vi "Main.vi"() -> ()   [LabVIEW 2020]
doc: "[Covers: REQ08]\n[Covers: REQ04]\n[Covers: REQ05]\n[Covers: REQ01]\n[Covers: REQ07]\n[Covers: REQ11]\n[Covers: REQ13]\n[Covers: REQ14]\n[Covers: REQ16]\n[Covers: REQ17]\n[Covers: REQ18]\n[Covers: REQ19]\n[Covers: REQ02]\n[Covers: REQ20]\n[Covers: REQ21]"
uses:
  TypeDef's/Estados - Consumidor.ctl
  TypeDef's/Dados consumidor.ctl
  <vilib>/Utility/sysdir.llb/System Directory Type.ctl
  <vilib>/Waveform/WDTOps.llb/WDT Append Waveforms DBL.vi
  <vilib>/Waveform/WDTOps.llb/WDT Waveform Duration DBL.vi
  <vilib>/measure/NI_MABase.lvlib
panel:
  in  "physical channels":tag
  in  "Canal físico":tag
  in  "Boolean 2":bool
  in  "Boolean":bool
  in  "Power":bool
  in  "Concatenar":bool
  in  "Adquirir entre cursores":bool
  in  "Deletar entre cursores":bool
  in  "Concatenar entre cursores":bool
  in  "Fase         º":dbl(slide) caption="Horizontal Slider" min=0.0 max=360.0 step=0.5 scale=0.0..360.0 scale format="%#.6g"
  in  "Offset":dbl(slide) caption="Vertical Slider" min=-10.0 max=10.0 step=0.01 scale=-10.0..10.0 scale format="%#2_2g"
  in  "Forma de onda":T1(ring) caption="Enum"
  in  "Tempo (Segundos)":dbl(knob)=1.0 min=0.0 max=1.0 step=0.01 scale=0.0..1.0
  in  "Abrir arquivo":bool
  in  "Salvar":bool
  out "Edição":waveform(dbl)(graph)
  out "Plot":waveform(dbl)(graph)
  in  "Razão cíclica (%)":dbl(knob)=50.0 min=0.0 max=100.0 step=0.5 scale=0.0..100.0
  in  "Amplitude":dbl(knob)=5.0 min=0.0 max=10.0 step=0.01 scale=0.0..10.0
  in  "Frequência":dbl(knob)=1.0 min=0.0 max=10.0 step=0.01 scale=0.0..10.0
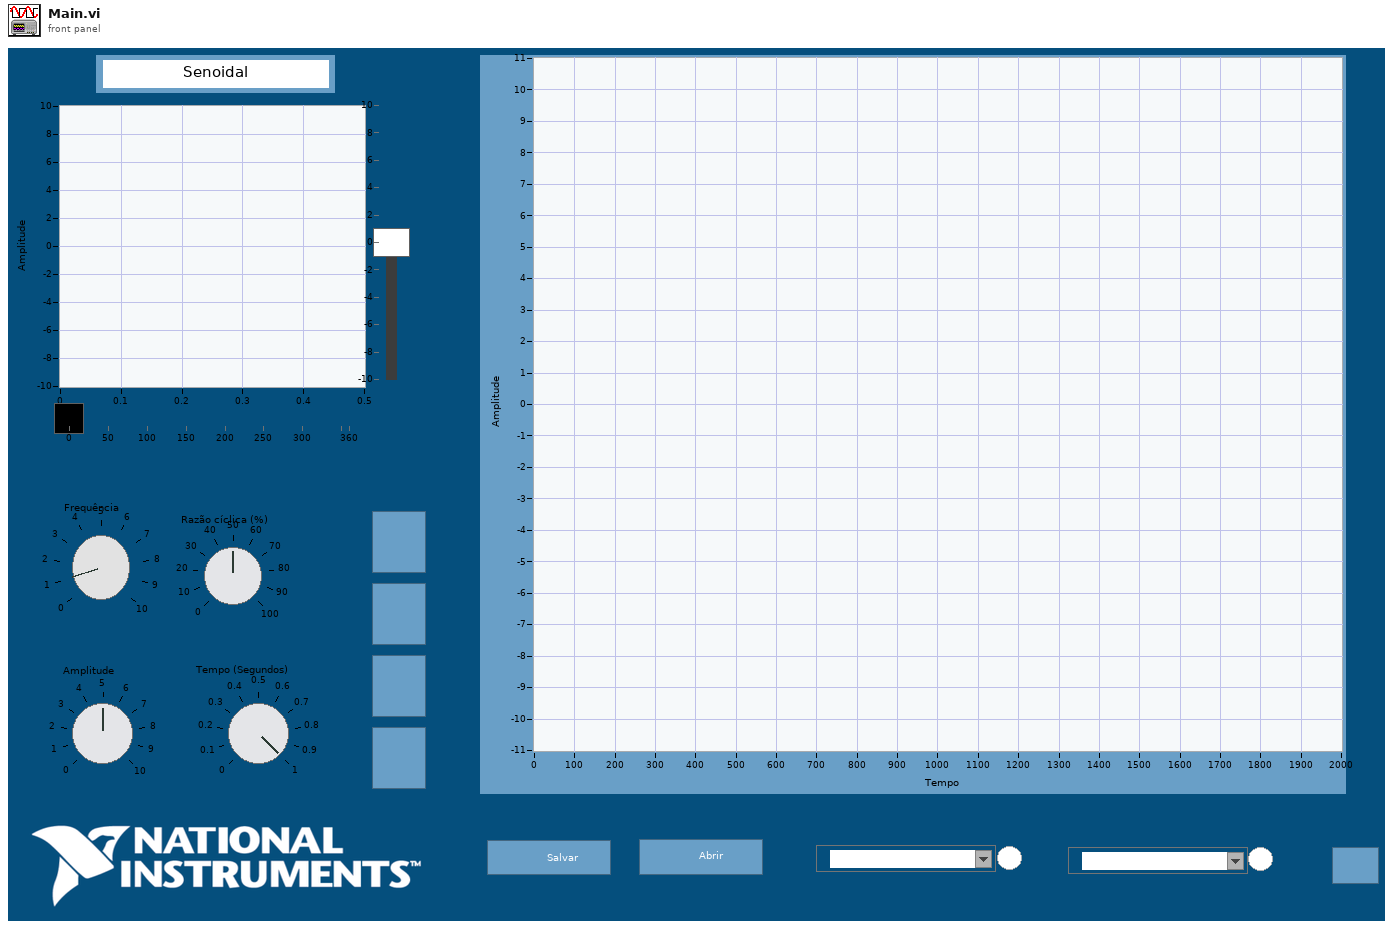
[diagram p1: front panel]
types:
  T1 = enum16{"Senoidal", "Triangular", "Quadrada", "Dente de Serra", "Trapezoidal"}
  T2 = enum16{"create", "fire - Simular onda", "fire - Editar onda", "fire - Salvar ou carregar onda", "destroy"}
  T3 = typedef "Estados - Consumidor.ctl" = enum16{"Gerar onda", "Inicialização", "Parada", "Plotar", "Concatenar", "Concatenar - Cursores", "Adquirir entre Cursores", "Deletar entre Cursores", "Salvar onda", "Carregar onda", "Posicionar Cursores", "Atualizar controles - Servidor", "Enviar onda - hardware", "Ler onda - hardware"}
  T4 = typedef "Dados consumidor.ctl" = cluster{"Onda gerada":cluster{"onda":waveform(dbl)}, "Onda modificada":cluster{"onda":waveform(dbl)}, "task out":refnum<k21>}
  T5 = typedef "Informações.ctl" = cluster{"Estados":T3, "Amplitude":dbl, "Informação\nde amostragem":cluster{"Fs":dbl, "#s":dbl}, "Frequência":dbl, "Offset":dbl, "Fase (Graus)":dbl, "Razão cíclica (%)":dbl, "Sinal":enum16{"Sine Wave", "Triangle Wave", "Square Wave", "Sawtooth Wave", "Trapezoidal Wave"}, "event registration refnum":refnum<event-registration>, "Posição Cursor 0":dbl, "Posição Cursor 1":dbl, "Flag Edição":i32}
  T6 = enum8{"Enabled", "Disabled", "Disabled and Grayed Out"}
  T7 = enum16{"Sine Wave", "Triangle Wave", "Square Wave", "Sawtooth Wave", "Trapezoidal Wave"}
  T8 = enum16{"open", "open or create", "create or replace", "create", "open (read-only)"}
  T9 = typedef "System Directory Type.ctl" = i32
  T10 = cluster{"Amostras / s":dbl, "Quantidade\nde amostras":dbl}
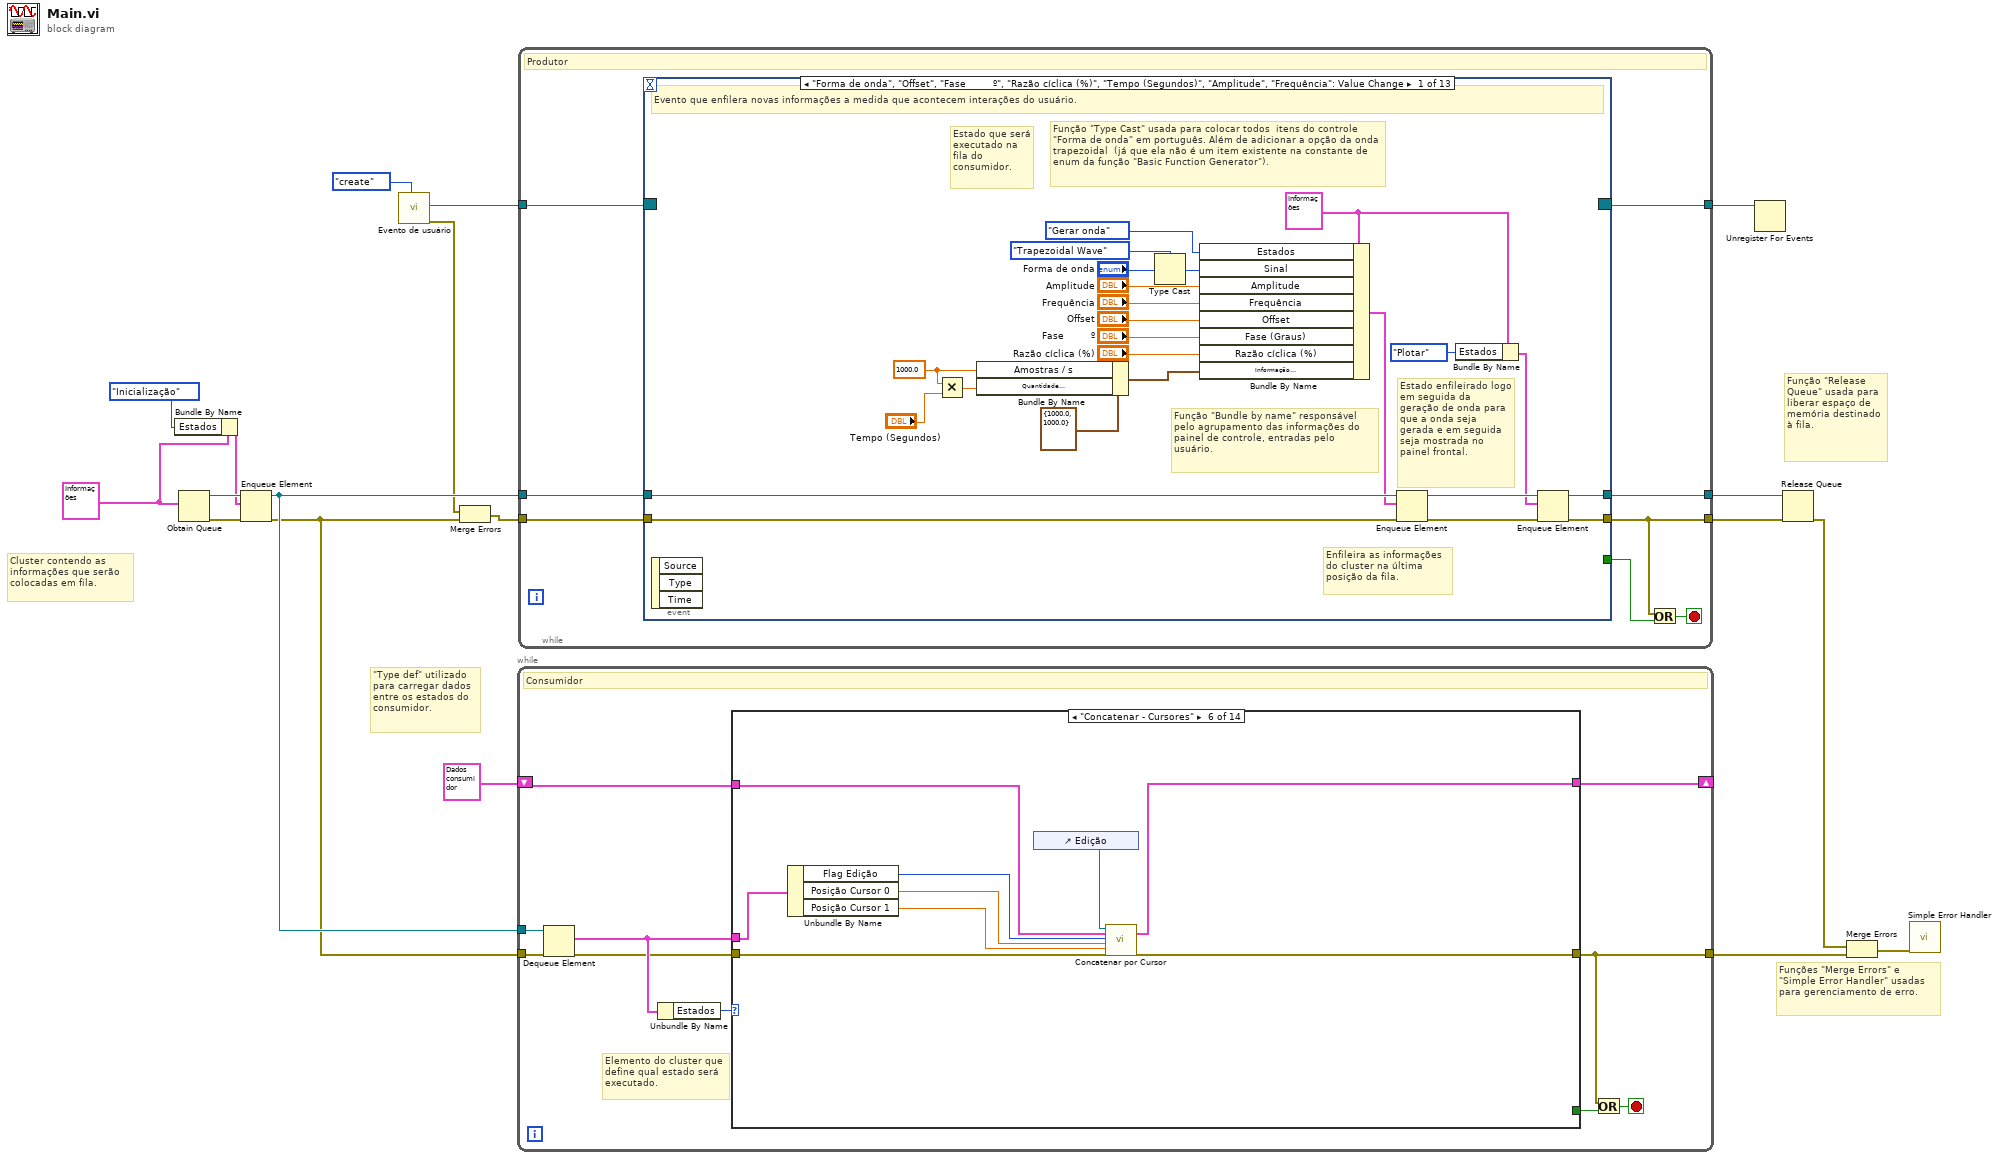
[diagram p0: block diagram]
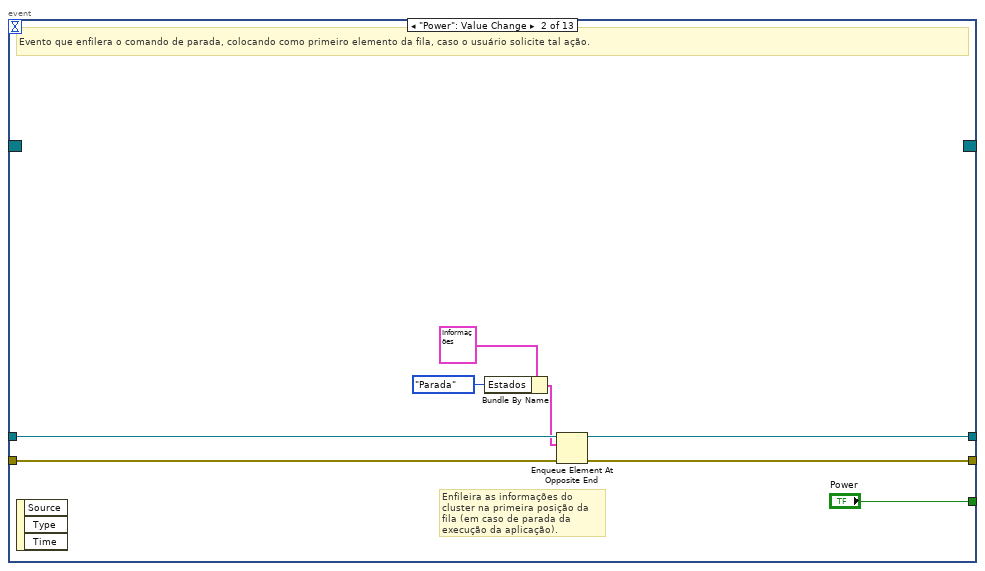
[diagram p2: hidden frame]
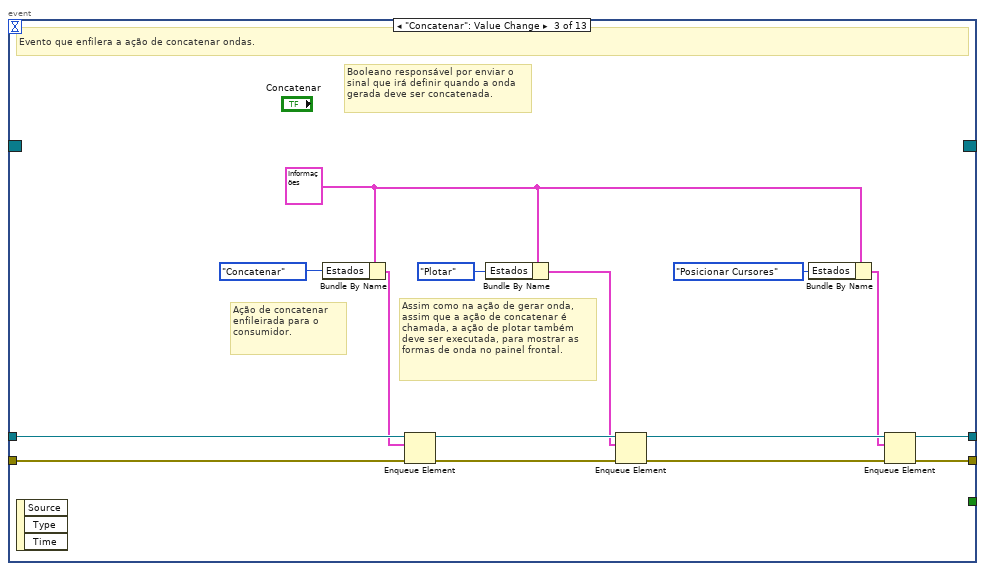
[diagram p3: hidden frame]
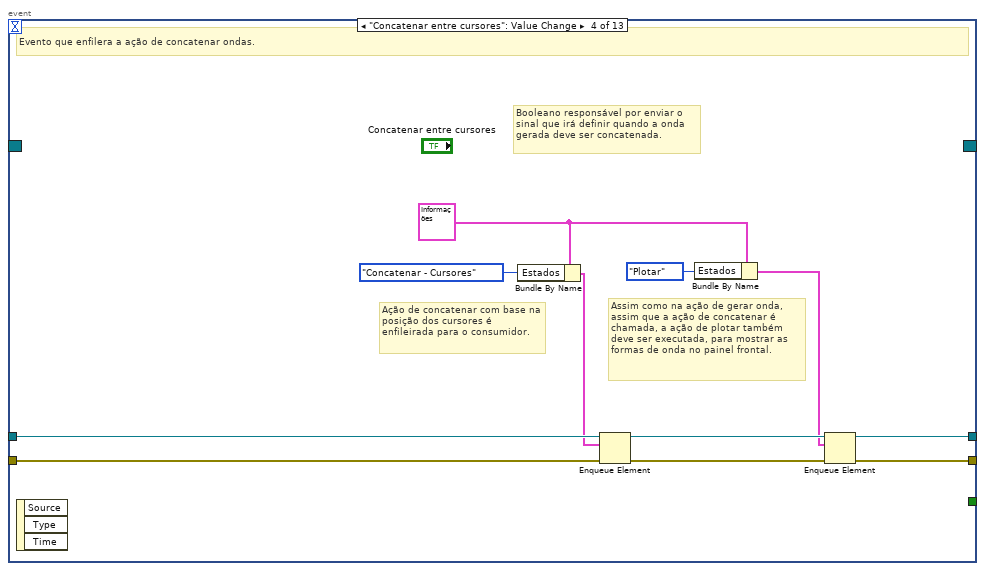
[diagram p4: hidden frame]
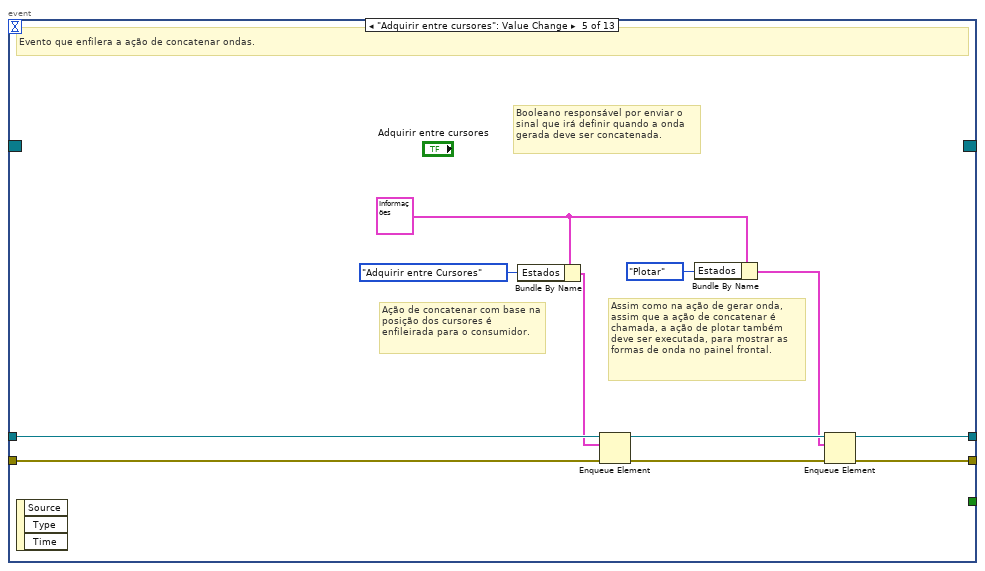
[diagram p5: hidden frame]
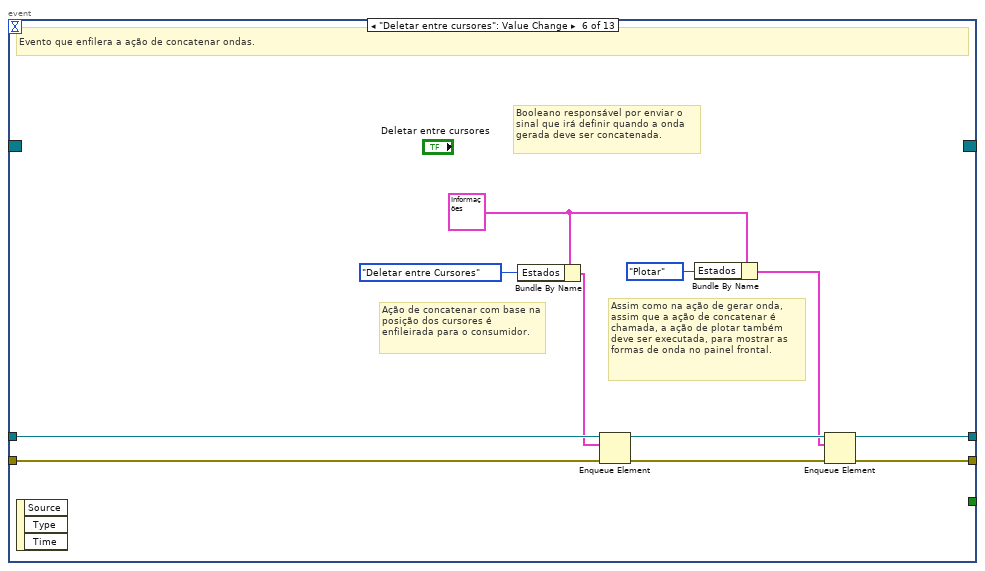
[diagram p6: hidden frame]
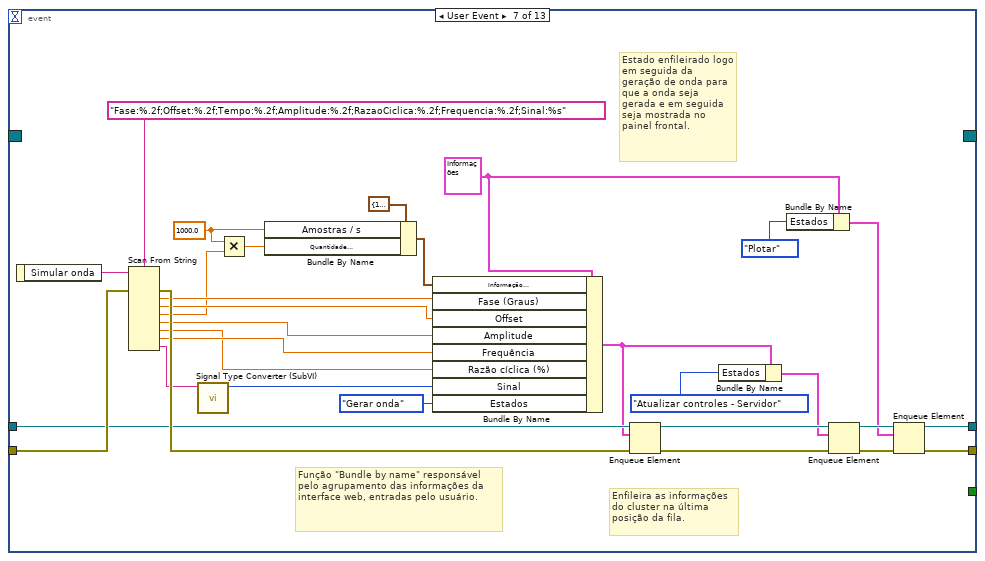
[diagram p7: hidden frame]
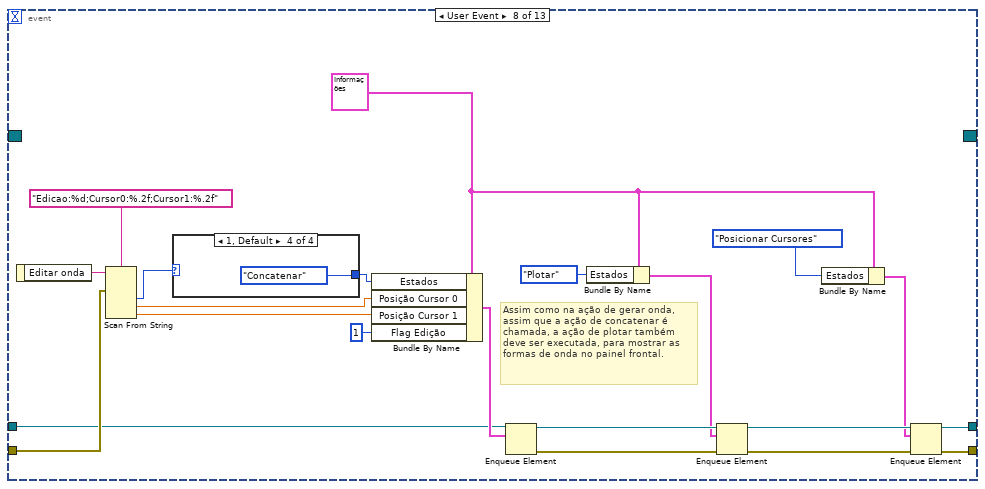
[diagram p8: hidden frame]
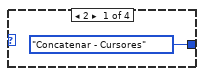
[diagram p9: hidden frame]
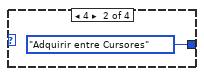
[diagram p10: hidden frame]
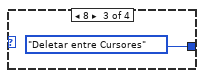
[diagram p11: hidden frame]
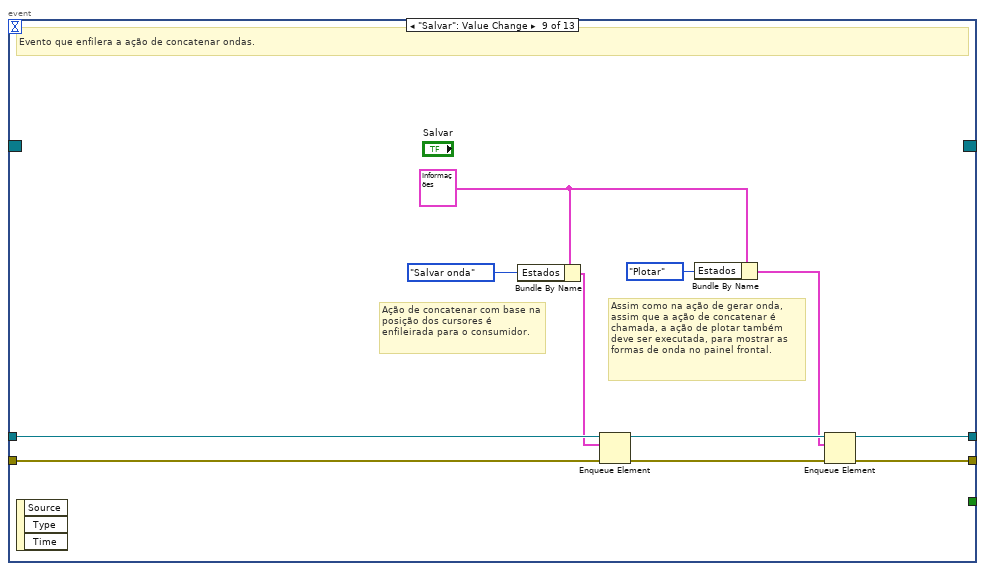
[diagram p12: hidden frame]
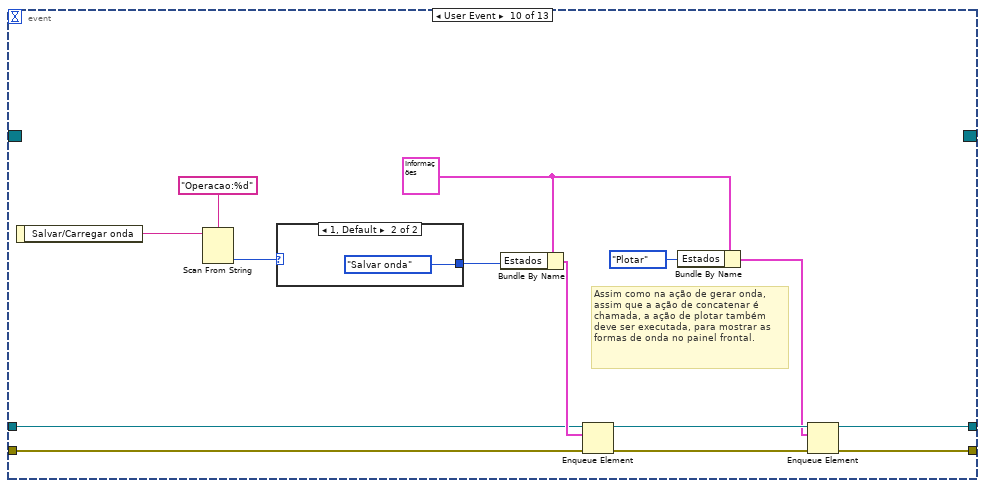
[diagram p13: hidden frame]
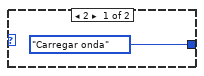
[diagram p14: hidden frame]
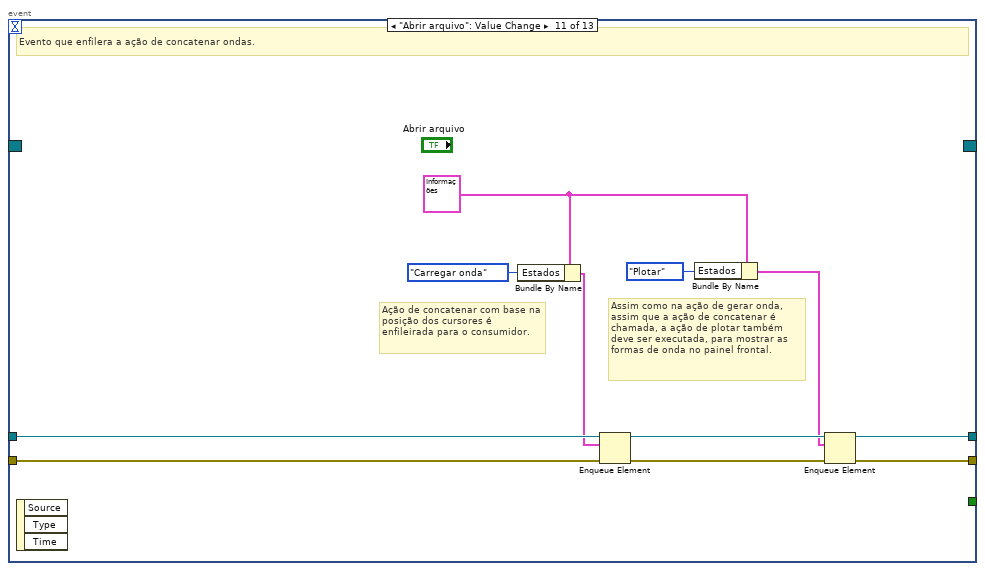
[diagram p15: hidden frame]
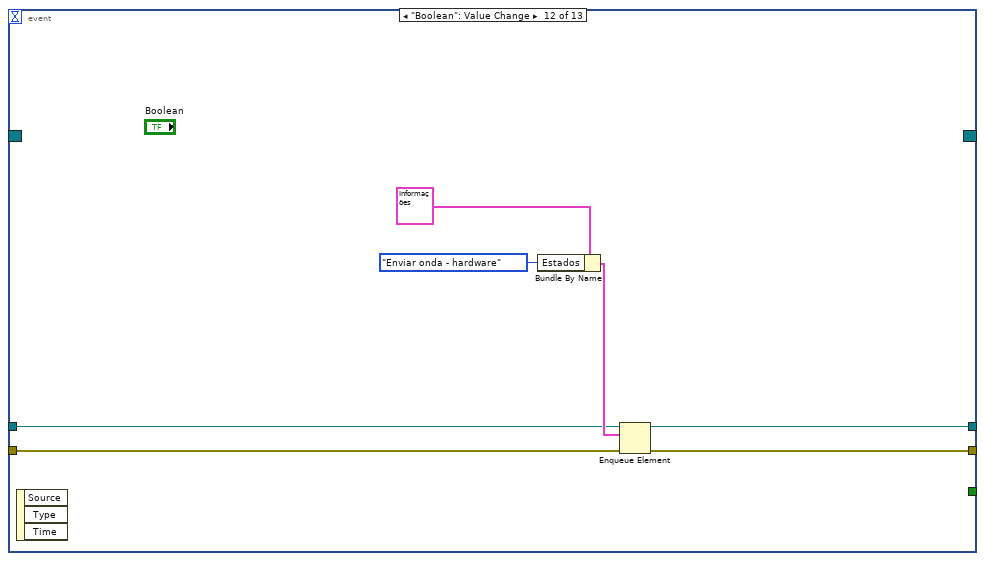
[diagram p16: hidden frame]
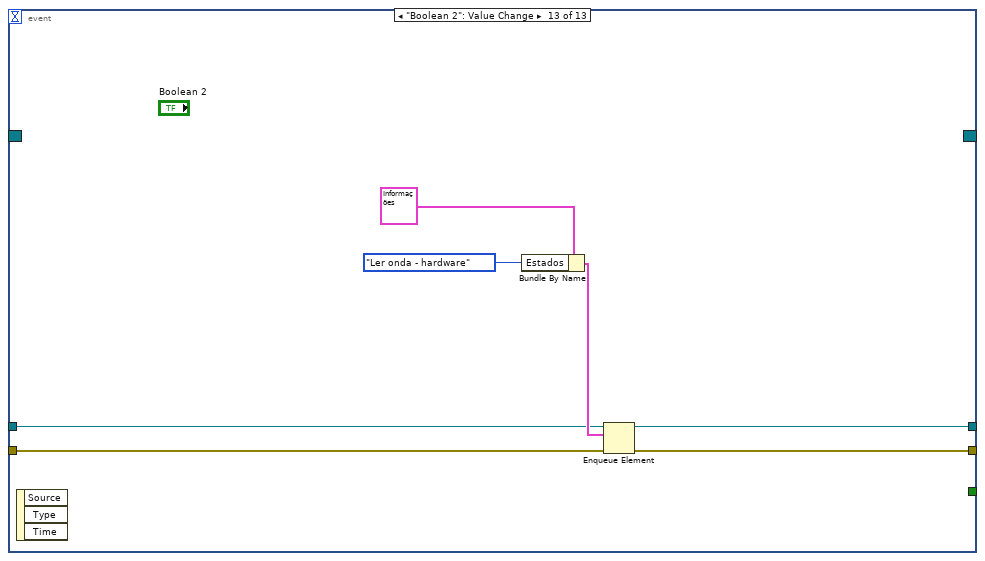
[diagram p17: hidden frame]
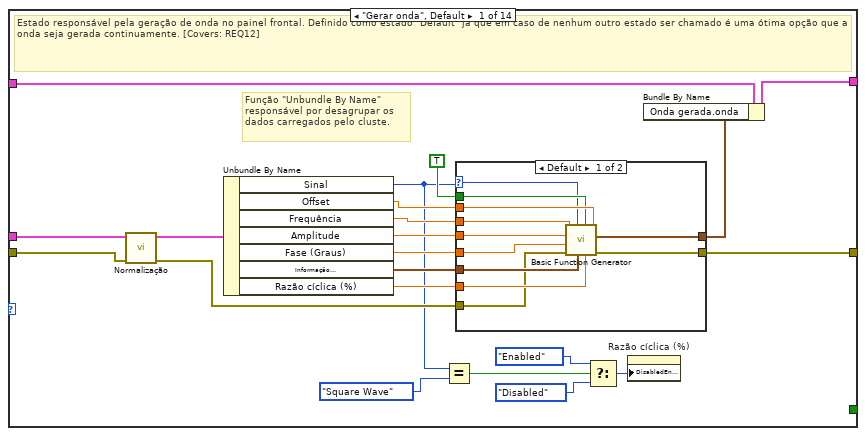
[diagram p18: hidden frame]
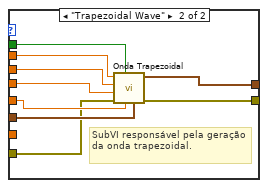
[diagram p19: hidden frame]
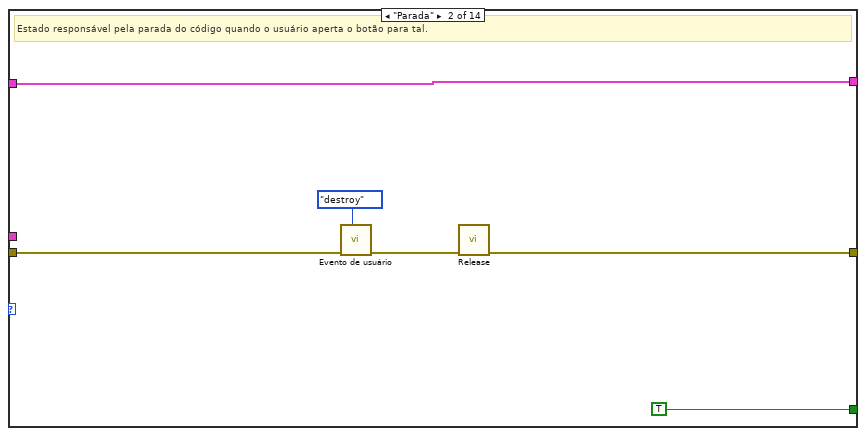
[diagram p20: hidden frame]
diagram:
  w7 = T5 {"Estados"=enum."Gerar onda", "Amplitude"=0.0, "Informação\nde amostragem"={"Fs"=1000.0, "#s"=1000.0}, "Frequência"=0.0, "Offset"=0.0, "Fase (Graus)"=0.0, "Razão cíclica (%)"=0.0, "Sinal"=enum."Sine Wave", "event registration refnum"=refnum, "Posição Cursor 0"=0.0, "Posição Cursor 1"=0.0, "Flag Edição"=0}
  # "\"Type def\" utilizado para carregar dados entre os estados do consumidor."
  # "Funções \"Merge Errors\" e \"Simple Error Handler\" usadas para gerenciamento de erro."
  # "Função \"Release Queue\" usada para liberar espaço de memória destinado à fila."
  # "Cluster contendo as informações que serão colocadas em fila."
  n1 = Bundle By Name(cluster=w7, "Estados"=Estados_-_Consumidor."Inicialização") -> (w9:T5)
  n2 = Obtain Queue(element data type=w7) -> (queue out=w11:refnum<queue>, error out=w13:errorcluster)  [unwired: 4 in, 1 out]
  n3 = Enqueue Element(queue=w11, element=w9, error in (no error)=w13) -> (queue out=w10:refnum<queue>, error out=w6:errorcluster)  [unwired: 1 in, 1 out]
  n4 = call "Evento de usuário.vi"("Enum"=T2."create") -> ("error out"=w4:errorcluster, "Event Registration Refnum"=w3:refnum<event-registration>)  [unwired: 9 in]
  n5 = Merge Errors(w4, w6) -> (w5:errorcluster)
  n6 = while {
    tunnel: w10 -> [w22]
    tunnel: [w19] -> w15
    tunnel: w6 -> [w23]
    shift-right: [w21] -> _
    shift-left: T4 {"Onda gerada"={"onda"={"t0"=timestamp(0 s since 1904-01-01), "dt"=1.0, "Y"=[]}}, "Onda modificada"={"onda"={"t0"=timestamp(0 s since 1904-01-01), "dt"=1.0, "Y"=[]}}, "task out"=""} ("Cluster 3") -> [w20]
    stop <- w25 stop-if-true
    # "Elemento do cluster que define qual estado será executado."
    # "Consumidor"
    n7 = Dequeue Element(queue=w22, error in (no error)=w23) -> (element=w27:T5, error out=w24:errorcluster)  [unwired: 1 in, 2 out]
    n8 = Unbundle By Name(w27) -> ("Estados"=w28:T3)
    n9 = case shown="\"Concatenar - Cursores\"" w28 {
      tunnel: w27 -> [w49 _ _ _ _ w101 w110 w119 _ _ _ w204 _ _]
      tunnel: [_ TRUE _ _ _ _ _ _ _ _ _ _ _ _] -> w26
      tunnel: [w41 w70 w77 w84 w91 w105 w112 w123 w131 w152 w185 w193 w206 w225] -> w19
      tunnel: w24 -> [w36 w73 w82 w87 w91 w106 w113 w124 w127 w155 w188 w193 w211 w228]
      tunnel: [w39 w74 w83 w89 w92 w104 w111 w122 w128 w153 w190 w205 w212 w220] -> w21
      tunnel: w20 -> [w40 w74 w83 w90 w92 w102 w114 w121 w132 w154 w190 w205 w212 w220]
      frame "Gerar onda", Default {
        # "Função \"Unbundle By Name\" responsável por desagrupar os dados carregados pelo cluste."
        # "Estado responsável pela geração de onda no painel frontal. Definido como estado \"Default\" já que em caso de nenhum outro estado ser chamado é uma ótima opção que a onda seja gerada continuamente. [Covers: REQ12]"
        n10 = call "Normalização.vi"("error in (no error)"=w36, 11:w49) -> ("error out"=w35:errorcluster, 3:w37:T5)  [unwired: 8 in]
        n11 = Unbundle By Name(w37) -> ("Sinal"=w29:T7, "Offset"=w48:dbl, "Frequência"=w47:dbl, "Amplitude"=w46:dbl, "Fase (Graus)"=w45:dbl, "Informação\nde amostragem"=w44:cluster{"Fs":dbl, "#s":dbl}, "Razão cíclica (%)"=w43:dbl)
        n12 = Equal?(x=w29, y=T7."Square Wave" ("Sinal")) -> (x = y?=w34:bool)
        n13 = case shown="Default" w29 {
          selector: w29 -> [w52 _]
          tunnel: w48 -> [w60 w63]
          tunnel: w47 -> [w59 w65]
          tunnel: w46 -> [w58 w64]
          tunnel: w45 -> [w57 w68]
          tunnel: w44 -> [w56 w67]
          tunnel: w43 -> [w55 _]
          tunnel: [w54 w66] -> w38
          tunnel: TRUE ("reset signal") -> [w53 w69]
          tunnel: [w51 w61] -> w41
          tunnel: w35 -> [w50 w62]
          frame Default {
            n14 = call <vilib>:"Basic Function Generator.vi"("offset"=w60, "square wave duty cycle (%)"=w55, "reset signal"=w53, "sampling info"=w56, "signal type"=w52, "error in (no error)"=w50, "phase"=w57, "amplitude"=w58, "frequency"=w59) -> ("error out"=w51:errorcluster, "signal out"=w54:waveform(dbl))  [unwired: 1 out]
          }
          frame "Trapezoidal Wave" {
            # "SubVI responsável pela geração da onda trapezoidal."
            n15 = call "Onda Trapezoidal.vi"("Informação\nde amostragem"=w67, "Fase (Graus)"=w68, "Reset do sinal"=w69, "Entrada de erro"=w62, "Amplitude"=w64, "Frequência"=w65, "Offset"=w63) -> ("Saída de erro"=w61:errorcluster, "Saída de sinal"=w66:waveform(dbl))  [unwired: 3 in]
          }
        }
        n16 = Select(t=T6."Enabled" ("Disabled"), s=w34, f=T6."Disabled" ("Disabled")) -> (s? t:f=w33:T6)
        n17 = property on="Razão cíclica (%)" class="Knob (strict)"("DisabledEnum"=w33) -> ()  [unwired: 2 in, 2 out]
        n18 = Bundle By Name(cluster=w40, "Onda gerada.onda"=w38) -> (w39:T4)
      }
      frame "Parada" {
        # "Estado responsável pela parada do código quando o usuário aperta o botão para tal."
        n19 = call "Evento de usuário.vi"("Enum"=T2."destroy", "error in (no error)"=w73) -> ("error out"=w71:errorcluster)  [unwired: 8 in, 1 out]
        n20 = call "Release.vi"("error in"=w71) -> ("error out"=w70:errorcluster)  [unwired: 10 in]
      }
      frame "Plotar" {
        # "FGV responsável por atualizar os dados da onda para envio para a interface web"
        # "Plot da onda editada pelo usuário."
        # "Plot da onda definida e gerada pelo usuário."
        # "Estado encarregado de exibir no painel frontal as formas de onda."
        n21 = Unbundle By Name(w83) -> ("Onda gerada.onda"=w81:waveform(dbl))
        "Plot" <- w81
        n22 = call "Plotar gráficos.vi"("Enum"=enum16{"set", "get"}."set", "error in (no error)"=w82, "Entrada Cluster de onda"=w81) -> ("error out"=w78:errorcluster)  [unwired: 7 in, 1 out]
        n23 = Unbundle By Name(w83) -> ("Onda modificada.onda"=w76:waveform(dbl))
        "Edição" <- w76
        n24 = call "Plotar gráfico edição.vi"("Enum"=enum16{"set", "get"}."set", "error in (no error)"=w78, "Entrada Cluster de onda"=w76) -> ("error out"=w77:errorcluster)  [unwired: 7 in, 1 out]
      }
      frame "Concatenar" {
        # "Função \"Append Waveforms\" utilizada para concatenar as ondas geradas desejadas."
        # "Estado encarregado de concatenar formas de onda de maneira sequencial."
        n25 = Unbundle By Name(w90) -> ("Onda modificada.onda"=w88:waveform(dbl), "Onda gerada.onda"=w86:waveform(dbl))
        n26 = call-poly <vilib>:"Append Waveforms.vi"("error in (no error)"=w87, "waveform B"=w86, "waveform A"=w88) -> ("error out"=w84:errorcluster, "waveform out"=w85:waveform(dbl))  [unwired: 7 in]
        n27 = Bundle By Name(cluster=w90, "Onda modificada.onda"=w85) -> (w89:T4)
      }
      frame "Inicialização" {
        n28 = invoke on="Plot" class="WFGraph (strict)" method="Reinit To Default"() -> ()  [unwired: 3 in, 3 out]
        n29 = property on="Razão cíclica (%)" class="Knob (strict)"("DisabledEnum"=T6."Disabled" ("Disabled")) -> ()  [unwired: 2 in, 2 out]
        n30 = invoke on="Tempo (Segundos)" class="Knob (strict)" method="Reinit To Default"() -> ()  [unwired: 3 in, 3 out]
        n31 = invoke on="Razão cíclica (%)" class="Knob (strict)" method="Reinit To Default"() -> ()  [unwired: 3 in, 3 out]
        n32 = invoke on="Edição" class="WFGraph (strict)" method="Reinit To Default"() -> ()  [unwired: 3 in, 3 out]
        n33 = property on="Edição" class="WFGraph (strict)"("Active Cursor"=u32 0, "Cursor.Visible"=FALSE, "Active Cursor"=u32 1, "Cursor.Visible"=FALSE) -> ()  [unwired: 2 in, 2 out]
        n34 = invoke on="Frequência" class="Knob (strict)" method="Reinit To Default"() -> ()  [unwired: 3 in, 3 out]
        n35 = invoke on="Amplitude" class="Knob (strict)" method="Reinit To Default"() -> ()  [unwired: 3 in, 3 out]
      }
      frame "Concatenar - Cursores" {
        n36 = Unbundle By Name(w101) -> ("Flag Edição"=w100:i32, "Posição Cursor 0"=w99:dbl, "Posição Cursor 1"=w98:dbl)
        n37 = control-ref of="Edição"() -> (w103:refnum<vi>)
        n38 = call "Concatenar por Cursor.vi"("WaveformGraph in"=w103, "Cluster 3"=w102, "Flag"=w100, "Cursor 0"=w99, "Cursor 1"=w98, "error in"=w106) -> ("output cluster"=w104:T4, "error out"=w105:errorcluster)  [unwired: 12 in]
      }
      frame "Adquirir entre Cursores" {
        n39 = Unbundle By Name(w110) -> ("Flag Edição"=w109:i32, "Posição Cursor 0"=w108:dbl, "Posição Cursor 1"=w107:dbl)
        n40 = control-ref of="Edição"() -> (w115:refnum<vi>)
        n41 = call "Adquirir entre cursores.vi"("WaveformGraph in"=w115, "Input Cluster"=w114, "Flag"=w109, "Cursor 0"=w108, "Cursor 1"=w107, "error in"=w113) -> ("Output Cluster"=w111:T4, "error out"=w112:errorcluster)  [unwired: 12 in]
      }
      frame "Deletar entre Cursores" {
        n42 = Unbundle By Name(w119) -> ("Flag Edição"=w118:i32, "Posição Cursor 0"=w117:dbl, "Posição Cursor 1"=w116:dbl)
        n43 = control-ref of="Edição"() -> (w120:refnum<vi>)
        n44 = call "Deletar entre Cursores.vi"("WaveformGraph in"=w120, "Cluster 3"=w121, "Flag"=w118, "Cursor 0"=w117, "Cursor 1"=w116, "error in"=w124) -> ("output cluster"=w122:T4, "error out"=w123:errorcluster)  [unwired: 12 in]
      }
      frame "Salvar onda" {
        w134 = T9 2 items=["User Home"=0, "User Desktop"=1, "User Documents"=2, "User Application Data"=3, "User Preferences"=4, "User Temporary"=5, "Public Documents"=6, "Public Application Data"=7, "Public Preferences"=8, "Public Cache"=13, "System Core Libraries"=9, "System Installed Libraries"=10, "Application Files"=11, "Boot Volume Root"=12] ("system directory type")
        n45 = call "Construção string (salvar).vi"("error in (no error)"=w127) -> ("error out"=w126:errorcluster, "String"=w125:string)  [unwired: 9 in]
        n46 = call <vilib>:"Get System Directory.vi"("system directory type"=w134) -> ("system directory"=w135:path)  [unwired: 10 in]
        n47 = call "File Dialog"("start path"=w135, "default name"=w125, "error in"=w126) -> ("selected path"=w133:path, "cancelled"=w130:bool, "error out"=w129:errorcluster)  [unwired: 9 in, 1 out]
        n48 = case shown="False" w130 {
          tunnel: w133 -> [w144 _]
          tunnel: w132 -> [w137 w150]
          tunnel: [w140 w147] -> w131
          tunnel: w129 -> [w138 w148]
          tunnel: [w137 w150] -> w128
          frame False {
            n49 = Unbundle By Name(w137) -> ("Onda modificada.onda"=w136:waveform(dbl))
            n50 = TDMS Open(5:FALSE ("create index file? (T)"), 8:w138, 10:T8."create" ("operation (0:open)"), 11:w144) -> (0:w143:errorcluster, 3:w142:refnum<k34>)  [unwired: 3 in]
            n51 = TDMS Write(0:w142, 9:w136, 11:w143) -> (4:w139:refnum<k34>, 15:w141:errorcluster)  [unwired: 3 in, 2 out]
            n52 = call "Set.vi"("Waveform In"=w136) -> ()  [unwired: 10 in, 1 out]
            n53 = TDMS Close(8:w141, 11:w139) -> (0:w140:errorcluster)  [unwired: 1 out]
          }
          frame True {
            n54 = call <vilib>:"Clear Errors.vi"("error in (no error)"=w148, "specific error code to clear (0: all)"=43) -> ("error out"=w147:errorcluster)  [unwired: 4 in, 1 out]
          }
        }
      }
      frame "Carregar onda" {
        w158 = T9 2 items=["User Home"=0, "User Desktop"=1, "User Documents"=2, "User Application Data"=3, "User Preferences"=4, "User Temporary"=5, "Public Documents"=6, "Public Application Data"=7, "Public Preferences"=8, "Public Cache"=13, "System Core Libraries"=9, "System Installed Libraries"=10, "Application Files"=11, "Boot Volume Root"=12] ("system directory type")
        n55 = call <vilib>:"Get System Directory.vi"("system directory type"=w158) -> ("system directory"=w159:path)  [unwired: 10 in]
        n56 = call "File Dialog2"("start path"=w159, "error in"=w155) -> ("selected path"=w156:path, "cancelled"=w151:bool, "error out"=w157:errorcluster)  [unwired: 10 in, 1 out]
        n57 = case shown="False" w151 {
          tunnel: w157 -> [w163 w183]
          tunnel: w156 -> [w171 _]
          tunnel: w154 -> [w167 w181]
          tunnel: [w166 w181] -> w153
          tunnel: [w164 w182] -> w152
          frame False {
            n58 = TDMS Open(5:FALSE ("create index file? (T)"), 8:w163, 10:T8."open (read-only)" ("operation (0:open)"), 11:w171) -> (0:w170:errorcluster, 3:w169:refnum<k34>)  [unwired: 3 in]
            n59 = TDMS Read(0:w169, 11:w170, 12:waveform(dbl) {"t0"=timestamp(0 s since 1904-01-01), "dt"=1.0, "Y"=[]} ("Onda modificada.onda")) -> (4:w168:refnum<k34>, 10:w162:waveform(dbl), 15:w161:errorcluster)  [unwired: 5 in, 3 out]
            n60 = Bundle By Name(cluster=w167, "Onda modificada.onda"=w162) -> (w166:T4)
            n61 = disable-structure shown="Enabled" {
              disable-tunnel: w162 -> [w177 w180]
              disable-tunnel: w161 -> [w176 w179]
              disable-tunnel: [w175 w178] -> w160
              frame Disabled {
                n62 = call "Plotar gráfico salvar e carregar onda.vi"("Enum"=enum16{"set", "get"}."set", "error in (no error)"=w176, "Entrada Cluster de onda"=w177) -> ("error out"=w175:errorcluster)  [unwired: 7 in, 1 out]
              }
              frame Enabled {
                n63 = call "Set.vi"("error in"=w179, "Waveform In"=w180) -> ("error out"=w178:errorcluster)  [unwired: 9 in]
              }
            }
            n64 = TDMS Close(8:w160, 11:w168) -> (0:w164:errorcluster)  [unwired: 1 out]
          }
          frame True {
            n65 = call <vilib>:"Clear Errors.vi"("error in (no error)"=w183, "specific error code to clear (0: all)"=43) -> ("error out"=w182:errorcluster)  [unwired: 4 in, 1 out]
          }
        }
      }
      frame "Posicionar Cursores" {
        n66 = Unbundle By Name(w190) -> ("Onda modificada.onda"=w189:waveform(dbl))
        n67 = call-poly <vilib>:"Waveform Duration.vi"("error in (no error)"=w188, "waveform in"=w189) -> ("error out"=w186:errorcluster, "duration"=w191:dbl)  [unwired: 7 in, 1 out]
        n68 = control-ref of="Edição"() -> (w187:refnum<vi>)
        n69 = call "Posicionamento de cursores.vi"("error in (no error)"=w186, "duration"=w191, "WaveformGraph in"=w187) -> ("error out"=w185:errorcluster)  [unwired: 8 in]
      }
      frame "Atualizar controles - Servidor" {
        # "Taxa de amostragem constante, sendo o mesmo valor numérico do evento de mudança de valor dos controles de geração de onda encontrado no Produtor (relação entre tempo, taxa de amostragem e número de amostras: T * Fs = #s ou T = #s / Fs)."
        # "Foi feito o processo inverso do encontrado no evento de mudança de controle no Produtor."
        n70 = Unbundle By Name(w204) -> ("Sinal"=w199:T7, "Fase (Graus)"=w203:dbl, "Offset"=w202:dbl, "Frequência"=w201:dbl, "Razão cíclica (%)"=w200:dbl, "Amplitude"=w192:dbl, "Informação\nde amostragem.#s"=w196:dbl)
        n71 = Divide(x=w196, y=1000.0) -> (x/y=w194:dbl)
        n72 = Type Cast(type=T1."Senoidal" ("Forma de onda 2"), x=w199) -> (*(type *) &x=w197:T1)
        n73 = property on="Fase         º" class="Slide (strict)"("Value"=w203) -> ()  [unwired: 2 in, 2 out]
        n74 = property on="Offset" class="Slide (strict)"("Value"=w202) -> ()  [unwired: 2 in, 2 out]
        n75 = property on="Frequência" class="Knob (strict)"("Value"=w201) -> ()  [unwired: 2 in, 2 out]
        n76 = property on="Razão cíclica (%)" class="Knob (strict)"("Value"=w200) -> ()  [unwired: 2 in, 2 out]
        n77 = property on="Amplitude" class="Knob (strict)"("Value"=w192) -> ()  [unwired: 2 in, 2 out]
        n78 = property on="Tempo (Segundos)" class="Knob (strict)"("Value"=w194) -> ()  [unwired: 2 in, 2 out]
        n79 = property on="Forma de onda" class="Enum (strict)"("Value"=w197) -> ()  [unwired: 2 in, 2 out]
      }
      frame "Enviar onda - hardware" {
        n80 = Unbundle By Name(w212) -> ("task out"=w208:refnum<k21>, "Onda modificada.onda"=w209:waveform(dbl))
        n81 = call "Voltage -Output.vi"("Entrada de erro"=w211, "Onda"=w209, "Canal físico"="Canal físico", "Task/Canal entrada"=w208) -> ("Saída de erro"=w207:errorcluster)  [unwired: 7 in]
        n82 = case shown="No Error" w207 {
          selector: w207 -> [w215 w217]
          tunnel: [w215 w216] -> w206
          frame No Error {
            n83 = One Button Dialog(message="Escrita em hardware realizada com sucesso!", button name ("OK")="OK") -> ()  [unwired: 1 out]
          }
          frame Error {
            n84 = call <vilib>:"Simple Error Handler.vi"("error in (no error)"=w217) -> ("error out"=w216:errorcluster)  [unwired: 4 in, 4 out]
          }
        }
      }
      frame "Ler onda - hardware" {
        n85 = Unbundle By Name(w220) -> ("Onda modificada.onda"=w219:waveform(dbl))
        n86 = call-poly <vilib>:"Waveform Duration.vi"("waveform in"=w219) -> ("duration"=w218:dbl)  [unwired: 8 in, 2 out]
        n87 = Open VI Reference(type specifier VI Refnum (for type only)=refnum<vi> refnum, vi path=path "C:/Users/lulima/Documents/Signal_Generator/Código/Servidor/SubVI's/Voltage input.vi", options=128, error in (no error)=w228) -> (vi reference=w222:refnum<vi>, error out=w227:errorcluster)  [unwired: 2 in]
        n88 = call-by-ref "Start Asynchronous Call"(reference=w222, error in=w227, "Y Scale.Range:Maximum"=w218, "physical channels"="physical channels") -> (error out=w225:errorcluster)  [unwired: 9 in, 2 out]
      }
    }
    n89 = Or(x=w19, y=w26) -> (x .or. y?=w25:bool)
  }
  n90 = while {
    tunnel: w10 -> [w236]
    tunnel: [w232] -> w18
    tunnel: w5 -> [w235]
    tunnel: [w231] -> w17
    tunnel: w3 -> [w230]
    tunnel: [w229] -> w2
    stop <- w233 stop-if-true
    # "Produtor"
    n91 = event shown="[0] \"Forma de onda\", \"Offset\", \"Fase         º\", \"Razão cíclica (%)\", \"Tempo (Segundos)\", \"Amplitude\", \"Frequência\": Value Change" {
      selector: w230 -> [_ _ _ _ _ _ _ _ _ _ _ _ _]
      dyn-events: [_ _ _ _ _ _ _ _ _ _ _ _ _] -> w229
      timeout: _ -> [_ _ _ _ _ _ _ _ _ _ _ _ _]
      tunnel: w236 -> [w260 w266 w281 w291 w302 w313 w335 w348 w379 w390 w406 w413 w419]
      tunnel: w235 -> [w259 w268 w283 w294 w305 w316 w345 w367 w382 w389 w409 w412 w420]
      tunnel: [w252 w267 w273 w292 w303 w314 w327 w350 w380 w387 w407 w410 w417] -> w231
      tunnel: [_ "Power" _ _ _ _ _ _ _ _ _ _ _] -> w234
      tunnel: [w250 w264 w272 w289 w300 w311 w329 w349 w377 w388 w404 w411 w418] -> w232
      event "Forma de onda", "Offset", "Fase         º", "Razão cíclica (%)", "Tempo (Segundos)", "Amplitude", "Frequência": Value Change {
        w239 = T5 {"Estados"=enum."Gerar onda", "Amplitude"=0.0, "Informação\nde amostragem"={"Fs"=1000.0, "#s"=1000.0}, "Frequência"=0.0, "Offset"=0.0, "Fase (Graus)"=0.0, "Razão cíclica (%)"=0.0, "Sinal"=enum."Sine Wave", "event registration refnum"=refnum, "Posição Cursor 0"=0.0, "Posição Cursor 1"=0.0, "Flag Edição"=0}
        w244 = 1000.0 ("Quantidade\nde amostras")
        # "Estado enfileirado logo em seguida da geração de onda para que a onda seja gerada e em seguida seja mostrada no painel frontal."
        # "Função \"Type Cast\" usada para colocar todos  itens do controle \"Forma de onda\" em português. Além de adicionar a opção da onda trapezoidal  (já que ela não é um item existente na constante de enum da função \"Basic Function Generator\")."
        # "Estado que será executado na fila do consumidor."
        # "Enfileira as informações do cluster na última posição da fila."
        # "Função \"Bundle by name\" responsável pelo agrupamento das informações do painel de controle, entradas pelo usuário."
        # "Evento que enfilera novas informações a medida que acontecem interações do usuário."
        n92 = event-data() -> ()  [unwired: 1 in, 3 out]
        n93 = Multiply(x=w244, y="Tempo (Segundos)") -> (x*y=w237:dbl)
        n94 = Bundle By Name(cluster=T10 {"Amostras / s"=1000.0, "Quantidade\nde amostras"=1000.0} ("Informação\nde amostragem"), "Amostras / s"=w244, "Quantidade\nde amostras"=w237) -> (w245:T10)
        n95 = Type Cast(type=T7."Trapezoidal Wave" ("Forma de onda"), x="Forma de onda") -> (*(type *) &x=w238:T7)
        n96 = Bundle By Name(cluster=w239, "Estados"=Estados_-_Consumidor."Gerar onda", "Sinal"=w238, "Amplitude"="Amplitude", "Frequência"="Frequência", "Offset"="Offset", "Fase (Graus)"="Fase         º", "Razão cíclica (%)"="Razão cíclica (%)", "Informação\nde amostragem"=w245) -> (w254:T5)
        n97 = Enqueue Element(queue=w260, element=w254, error in (no error)=w259) -> (queue out=w251:refnum<queue>, error out=w258:errorcluster)  [unwired: 1 in, 1 out]
        n98 = Bundle By Name(cluster=w239, "Estados"=Estados_-_Consumidor."Plotar") -> (w249:T5)
        n99 = Enqueue Element(queue=w251, element=w249, error in (no error)=w258) -> (queue out=w250:refnum<queue>, error out=w252:errorcluster)  [unwired: 1 in, 1 out]
      }
      event "Power": Value Change {
        # "Enfileira as informações do cluster na primeira posição da fila (em caso de parada da execução da aplicação)."
        # "Evento que enfilera o comando de parada, colocando como primeiro elemento da fila, caso o usuário solicite tal ação."
        n100 = event-data() -> ()  [unwired: 1 in, 3 out]
        n101 = Bundle By Name(cluster=T5 {"Estados"=enum."Gerar onda", "Amplitude"=0.0, "Informação\nde amostragem"={"Fs"=1000.0, "#s"=1000.0}, "Frequência"=0.0, "Offset"=0.0, "Fase (Graus)"=0.0, "Razão cíclica (%)"=0.0, "Sinal"=enum."Sine Wave", "event registration refnum"=refnum, "Posição Cursor 0"=0.0, "Posição Cursor 1"=0.0, "Flag Edição"=0}, "Estados"=Estados_-_Consumidor."Parada") -> (w265:T5)
        n102 = Enqueue Element At Opposite End(queue=w266, element=w265, error in (no error)=w268) -> (queue out=w264:refnum<queue>, error out=w267:errorcluster)  [unwired: 1 in, 1 out]
      }
      event "Concatenar": Value Change {
        w271 = T5 {"Estados"=enum."Gerar onda", "Amplitude"=0.0, "Informação\nde amostragem"={"Fs"=1000.0, "#s"=1000.0}, "Frequência"=0.0, "Offset"=0.0, "Fase (Graus)"=0.0, "Razão cíclica (%)"=0.0, "Sinal"=enum."Sine Wave", "event registration refnum"=refnum, "Posição Cursor 0"=0.0, "Posição Cursor 1"=0.0, "Flag Edição"=0}
        # "Assim como na ação de gerar onda, assim que a ação de concatenar é chamada, a ação de plotar também deve ser executada, para mostrar as formas de onda no painel frontal."
        # "Ação de concatenar enfileirada para o consumidor."
        # "Booleano responsável por enviar o sinal que irá definir quando a onda gerada deve ser concatenada."
        # "Evento que enfilera a ação de concatenar ondas."
        n103 = event-data() -> ()  [unwired: 1 in, 3 out]
        n104 = Bundle By Name(cluster=w271, "Estados"=Estados_-_Consumidor."Concatenar") -> (w279:T5)
        n105 = Enqueue Element(queue=w281, element=w279, error in (no error)=w283) -> (queue out=w280:refnum<queue>, error out=w282:errorcluster)  [unwired: 1 in, 1 out]
        n106 = Bundle By Name(cluster=w271, "Estados"=Estados_-_Consumidor."Plotar") -> (w278:T5)
        n107 = Enqueue Element(queue=w280, element=w278, error in (no error)=w282) -> (queue out=w275:refnum<queue>, error out=w274:errorcluster)  [unwired: 1 in, 1 out]
        n108 = Bundle By Name(cluster=w271, "Estados"=Estados_-_Consumidor."Posicionar Cursores") -> (w269:T5)
        n109 = Enqueue Element(queue=w275, element=w269, error in (no error)=w274) -> (queue out=w272:refnum<queue>, error out=w273:errorcluster)  [unwired: 1 in, 1 out]
      }
      event "Concatenar entre cursores": Value Change {
        w284 = T5 {"Estados"=enum."Gerar onda", "Amplitude"=0.0, "Informação\nde amostragem"={"Fs"=1000.0, "#s"=1000.0}, "Frequência"=0.0, "Offset"=0.0, "Fase (Graus)"=0.0, "Razão cíclica (%)"=0.0, "Sinal"=enum."Sine Wave", "event registration refnum"=refnum, "Posição Cursor 0"=0.0, "Posição Cursor 1"=0.0, "Flag Edição"=0}
        # "Assim como na ação de gerar onda, assim que a ação de concatenar é chamada, a ação de plotar também deve ser executada, para mostrar as formas de onda no painel frontal."
        # "Ação de concatenar com base na posição dos cursores é enfileirada para o consumidor."
        # "Booleano responsável por enviar o sinal que irá definir quando a onda gerada deve ser concatenada."
        # "Evento que enfilera a ação de concatenar ondas."
        n110 = event-data() -> ()  [unwired: 1 in, 3 out]
        n111 = Bundle By Name(cluster=w284, "Estados"=Estados_-_Consumidor."Concatenar - Cursores") -> (w288:T5)
        n112 = Enqueue Element(queue=w291, element=w288, error in (no error)=w294) -> (queue out=w290:refnum<queue>, error out=w293:errorcluster)  [unwired: 1 in, 1 out]
        n113 = Bundle By Name(cluster=w284, "Estados"=Estados_-_Consumidor."Plotar") -> (w287:T5)
        n114 = Enqueue Element(queue=w290, element=w287, error in (no error)=w293) -> (queue out=w289:refnum<queue>, error out=w292:errorcluster)  [unwired: 1 in, 1 out]
      }
      event "Adquirir entre cursores": Value Change {
        w295 = T5 {"Estados"=enum."Gerar onda", "Amplitude"=0.0, "Informação\nde amostragem"={"Fs"=1000.0, "#s"=1000.0}, "Frequência"=0.0, "Offset"=0.0, "Fase (Graus)"=0.0, "Razão cíclica (%)"=0.0, "Sinal"=enum."Sine Wave", "event registration refnum"=refnum, "Posição Cursor 0"=0.0, "Posição Cursor 1"=0.0, "Flag Edição"=0}
        # "Assim como na ação de gerar onda, assim que a ação de concatenar é chamada, a ação de plotar também deve ser executada, para mostrar as formas de onda no painel frontal."
        # "Ação de concatenar com base na posição dos cursores é enfileirada para o consumidor."
        # "Booleano responsável por enviar o sinal que irá definir quando a onda gerada deve ser concatenada."
        # "Evento que enfilera a ação de concatenar ondas."
        n115 = event-data() -> ()  [unwired: 1 in, 3 out]
        n116 = Bundle By Name(cluster=w295, "Estados"=Estados_-_Consumidor."Adquirir entre Cursores") -> (w299:T5)
        n117 = Enqueue Element(queue=w302, element=w299, error in (no error)=w305) -> (queue out=w301:refnum<queue>, error out=w304:errorcluster)  [unwired: 1 in, 1 out]
        n118 = Bundle By Name(cluster=w295, "Estados"=Estados_-_Consumidor."Plotar") -> (w298:T5)
        n119 = Enqueue Element(queue=w301, element=w298, error in (no error)=w304) -> (queue out=w300:refnum<queue>, error out=w303:errorcluster)  [unwired: 1 in, 1 out]
      }
      event "Deletar entre cursores": Value Change {
        w306 = T5 {"Estados"=enum."Gerar onda", "Amplitude"=0.0, "Informação\nde amostragem"={"Fs"=1000.0, "#s"=1000.0}, "Frequência"=0.0, "Offset"=0.0, "Fase (Graus)"=0.0, "Razão cíclica (%)"=0.0, "Sinal"=enum."Sine Wave", "event registration refnum"=refnum, "Posição Cursor 0"=0.0, "Posição Cursor 1"=0.0, "Flag Edição"=0}
        # "Assim como na ação de gerar onda, assim que a ação de concatenar é chamada, a ação de plotar também deve ser executada, para mostrar as formas de onda no painel frontal."
        # "Ação de concatenar com base na posição dos cursores é enfileirada para o consumidor."
        # "Booleano responsável por enviar o sinal que irá definir quando a onda gerada deve ser concatenada."
        # "Evento que enfilera a ação de concatenar ondas."
        n120 = event-data() -> ()  [unwired: 1 in, 3 out]
        n121 = Bundle By Name(cluster=w306, "Estados"=Estados_-_Consumidor."Deletar entre Cursores") -> (w310:T5)
        n122 = Enqueue Element(queue=w313, element=w310, error in (no error)=w316) -> (queue out=w312:refnum<queue>, error out=w315:errorcluster)  [unwired: 1 in, 1 out]
        n123 = Bundle By Name(cluster=w306, "Estados"=Estados_-_Consumidor."Plotar") -> (w309:T5)
        n124 = Enqueue Element(queue=w312, element=w309, error in (no error)=w315) -> (queue out=w311:refnum<queue>, error out=w314:errorcluster)  [unwired: 1 in, 1 out]
      }
      event User Event {
        w326 = T5 {"Estados"=enum."Gerar onda", "Amplitude"=0.0, "Informação\nde amostragem"={"Fs"=1000.0, "#s"=1000.0}, "Frequência"=0.0, "Offset"=0.0, "Fase (Graus)"=0.0, "Razão cíclica (%)"=0.0, "Sinal"=enum."Sine Wave", "event registration refnum"=refnum, "Posição Cursor 0"=0.0, "Posição Cursor 1"=0.0, "Flag Edição"=0}
        w341 = 1000.0 ("Quantidade\nde amostras")
        # "Estado enfileirado logo em seguida da geração de onda para que a onda seja gerada e em seguida seja mostrada no painel frontal."
        # "Enfileira as informações do cluster na última posição da fila."
        # "Função \"Bundle by name\" responsável pelo agrupamento das informações da interface web, entradas pelo usuário."
        n125 = event-data() -> ("Simular onda"=w344:string)  [unwired: 1 in]
        n126 = Scan From String(format string="Fase:%.2f;Offset:%.2f;Tempo:%.2f;Amplitude:%.2f;RazaoCiclica:%.2f;Frequencia:%.2f;Sinal:%s", input string=w344, error in=w345) -> (error out=w336:errorcluster, output 1=w333:dbl, output 2=w332:dbl, output 3=w331:dbl, output 4=w322:dbl, output 5=w320:dbl, output 6=w323:dbl, output 7=w321:string)  [unwired: 8 in, 2 out]
        n127 = call "Signal Type Converter (SubVI).vi"("Signal Type"=w321) -> ("Signal Type Out"=w319:T7)  [unwired: 10 in]
        n128 = Multiply(x=w341, y=w331) -> (x*y=w342:dbl)
        n129 = Bundle By Name(cluster=T10 {"Amostras / s"=1000.0, "Quantidade\nde amostras"=1000.0} ("Informação\nde amostragem"), "Amostras / s"=w341, "Quantidade\nde amostras"=w342) -> (w340:T10)
        n130 = Bundle By Name(cluster=w326, "Informação\nde amostragem"=w340, "Fase (Graus)"=w333, "Offset"=w332, "Amplitude"=w322, "Frequência"=w323, "Razão cíclica (%)"=w320, "Sinal"=w319, "Estados"=Estados_-_Consumidor."Gerar onda") -> (w317:T5)
        n131 = Enqueue Element(queue=w335, element=w317, error in (no error)=w336) -> (queue out=w338:refnum<queue>, error out=w339:errorcluster)  [unwired: 1 in, 1 out]
        n132 = Bundle By Name(cluster=w317, "Estados"=Estados_-_Consumidor."Atualizar controles - Servidor") -> (w337:T5)
        n133 = Bundle By Name(cluster=w326, "Estados"=Estados_-_Consumidor."Plotar") -> (w324:T5)
        n134 = Enqueue Element(queue=w338, element=w337, error in (no error)=w339) -> (queue out=w330:refnum<queue>, error out=w328:errorcluster)  [unwired: 1 in, 1 out]
        n135 = Enqueue Element(queue=w330, element=w324, error in (no error)=w328) -> (queue out=w329:refnum<queue>, error out=w327:errorcluster)  [unwired: 1 in, 1 out]
      }
      event User Event {
        w353 = T5 {"Estados"=enum."Gerar onda", "Amplitude"=0.0, "Informação\nde amostragem"={"Fs"=1000.0, "#s"=1000.0}, "Frequência"=0.0, "Offset"=0.0, "Fase (Graus)"=0.0, "Razão cíclica (%)"=0.0, "Sinal"=enum."Sine Wave", "event registration refnum"=refnum, "Posição Cursor 0"=0.0, "Posição Cursor 1"=0.0, "Flag Edição"=0}
        # "Assim como na ação de gerar onda, assim que a ação de concatenar é chamada, a ação de plotar também deve ser executada, para mostrar as formas de onda no painel frontal."
        n136 = event-data() -> ("Editar onda"=w366:string)  [unwired: 1 in]
        n137 = Scan From String(format string="Edicao:%d;Cursor0:%.2f;Cursor1:%.2f", input string=w366, error in=w367) -> (output 1=w357:i32, output 2=w355:dbl, output 3=w354:dbl)  [unwired: 4 in, 3 out]
        n138 = case shown="1, Default" w357 {
          tunnel: [Estados_-_Consumidor."Concatenar - Cursores" ("Estados") Estados_-_Consumidor."Adquirir entre Cursores" ("Estados") Estados_-_Consumidor."Deletar entre Cursores" ("Estados") Estados_-_Consumidor."Concatenar" ("Estados")] -> w362
          frame 2 {
          }
          frame 4 {
          }
          frame 8 {
          }
          frame 1, Default {
          }
        }
        n139 = Bundle By Name(cluster=w353, "Estados"=w362, "Posição Cursor 0"=w355, "Posição Cursor 1"=w354, "Flag Edição"=1) -> (w363:T5)
        n140 = Enqueue Element(queue=w348, element=w363) -> (queue out=w364:refnum<queue>, error out=w365:errorcluster)  [unwired: 2 in, 1 out]
        n141 = Bundle By Name(cluster=w353, "Estados"=Estados_-_Consumidor."Plotar") -> (w351:T5)
        n142 = Enqueue Element(queue=w364, element=w351, error in (no error)=w365) -> (queue out=w361:refnum<queue>, error out=w360:errorcluster)  [unwired: 1 in, 1 out]
        n143 = Bundle By Name(cluster=w353, "Estados"=Estados_-_Consumidor."Posicionar Cursores") -> (w347:T5)
        n144 = Enqueue Element(queue=w361, element=w347, error in (no error)=w360) -> (queue out=w349:refnum<queue>, error out=w350:errorcluster)  [unwired: 1 in, 1 out]
      }
      event "Salvar": Value Change {
        w372 = T5 {"Estados"=enum."Gerar onda", "Amplitude"=0.0, "Informação\nde amostragem"={"Fs"=1000.0, "#s"=1000.0}, "Frequência"=0.0, "Offset"=0.0, "Fase (Graus)"=0.0, "Razão cíclica (%)"=0.0, "Sinal"=enum."Sine Wave", "event registration refnum"=refnum, "Posição Cursor 0"=0.0, "Posição Cursor 1"=0.0, "Flag Edição"=0}
        # "Assim como na ação de gerar onda, assim que a ação de concatenar é chamada, a ação de plotar também deve ser executada, para mostrar as formas de onda no painel frontal."
        # "Ação de concatenar com base na posição dos cursores é enfileirada para o consumidor."
        # "Evento que enfilera a ação de concatenar ondas."
        n145 = event-data() -> ()  [unwired: 1 in, 3 out]
        n146 = Bundle By Name(cluster=w372, "Estados"=Estados_-_Consumidor."Salvar onda") -> (w376:T5)
        n147 = Enqueue Element(queue=w379, element=w376, error in (no error)=w382) -> (queue out=w378:refnum<queue>, error out=w381:errorcluster)  [unwired: 1 in, 1 out]
        n148 = Bundle By Name(cluster=w372, "Estados"=Estados_-_Consumidor."Plotar") -> (w375:T5)
        n149 = Enqueue Element(queue=w378, element=w375, error in (no error)=w381) -> (queue out=w377:refnum<queue>, error out=w380:errorcluster)  [unwired: 1 in, 1 out]
      }
      event User Event {
        w391 = T5 {"Estados"=enum."Gerar onda", "Amplitude"=0.0, "Informação\nde amostragem"={"Fs"=1000.0, "#s"=1000.0}, "Frequência"=0.0, "Offset"=0.0, "Fase (Graus)"=0.0, "Razão cíclica (%)"=0.0, "Sinal"=enum."Sine Wave", "event registration refnum"=refnum, "Posição Cursor 0"=0.0, "Posição Cursor 1"=0.0, "Flag Edição"=0}
        # "Assim como na ação de gerar onda, assim que a ação de concatenar é chamada, a ação de plotar também deve ser executada, para mostrar as formas de onda no painel frontal."
        n150 = event-data() -> ("Salvar/Carregar onda"=w385:string)  [unwired: 1 in]
        n151 = Scan From String(format string="Operacao:%d", input string=w385) -> (output 1=w386:i32)  [unwired: 3 in, 3 out]
        n152 = case shown="1, Default" w386 {
          tunnel: [Estados_-_Consumidor."Carregar onda" ("Estados") Estados_-_Consumidor."Salvar onda" ("Estados")] -> w383
          frame 2 {
          }
          frame 1, Default {
          }
        }
        n153 = Bundle By Name(cluster=w391, "Estados"=w383) -> (w394:T5)
        n154 = Enqueue Element(queue=w390, element=w394, error in (no error)=w389) -> (queue out=w395:refnum<queue>, error out=w396:errorcluster)  [unwired: 1 in, 1 out]
        n155 = Bundle By Name(cluster=w391, "Estados"=Estados_-_Consumidor."Plotar") -> (w393:T5)
        n156 = Enqueue Element(queue=w395, element=w393, error in (no error)=w396) -> (queue out=w388:refnum<queue>, error out=w387:errorcluster)  [unwired: 1 in, 1 out]
      }
      event "Abrir arquivo": Value Change {
        w399 = T5 {"Estados"=enum."Gerar onda", "Amplitude"=0.0, "Informação\nde amostragem"={"Fs"=1000.0, "#s"=1000.0}, "Frequência"=0.0, "Offset"=0.0, "Fase (Graus)"=0.0, "Razão cíclica (%)"=0.0, "Sinal"=enum."Sine Wave", "event registration refnum"=refnum, "Posição Cursor 0"=0.0, "Posição Cursor 1"=0.0, "Flag Edição"=0}
        # "Assim como na ação de gerar onda, assim que a ação de concatenar é chamada, a ação de plotar também deve ser executada, para mostrar as formas de onda no painel frontal."
        # "Ação de concatenar com base na posição dos cursores é enfileirada para o consumidor."
        # "Evento que enfilera a ação de concatenar ondas."
        n157 = event-data() -> ()  [unwired: 1 in, 3 out]
        n158 = Bundle By Name(cluster=w399, "Estados"=Estados_-_Consumidor."Carregar onda") -> (w403:T5)
        n159 = Enqueue Element(queue=w406, element=w403, error in (no error)=w409) -> (queue out=w405:refnum<queue>, error out=w408:errorcluster)  [unwired: 1 in, 1 out]
        n160 = Bundle By Name(cluster=w399, "Estados"=Estados_-_Consumidor."Plotar") -> (w402:T5)
        n161 = Enqueue Element(queue=w405, element=w402, error in (no error)=w408) -> (queue out=w404:refnum<queue>, error out=w407:errorcluster)  [unwired: 1 in, 1 out]
      }
      event "Boolean": Value Change {
        n162 = event-data() -> ()  [unwired: 1 in, 3 out]
        n163 = Bundle By Name(cluster=T5 {"Estados"=enum."Gerar onda", "Amplitude"=0.0, "Informação\nde amostragem"={"Fs"=1000.0, "#s"=1000.0}, "Frequência"=0.0, "Offset"=0.0, "Fase (Graus)"=0.0, "Razão cíclica (%)"=0.0, "Sinal"=enum."Sine Wave", "event registration refnum"=refnum, "Posição Cursor 0"=0.0, "Posição Cursor 1"=0.0, "Flag Edição"=0}, "Estados"=Estados_-_Consumidor."Enviar onda - hardware") -> (w416:T5)
        n164 = Enqueue Element(queue=w413, element=w416, error in (no error)=w412) -> (queue out=w411:refnum<queue>, error out=w410:errorcluster)  [unwired: 1 in, 1 out]
      }
      event "Boolean 2": Value Change {
        n165 = event-data() -> ()  [unwired: 1 in, 3 out]
        n166 = Bundle By Name(cluster=T5 {"Estados"=enum."Gerar onda", "Amplitude"=0.0, "Informação\nde amostragem"={"Fs"=1000.0, "#s"=1000.0}, "Frequência"=0.0, "Offset"=0.0, "Fase (Graus)"=0.0, "Razão cíclica (%)"=0.0, "Sinal"=enum."Sine Wave", "event registration refnum"=refnum, "Posição Cursor 0"=0.0, "Posição Cursor 1"=0.0, "Flag Edição"=0}, "Estados"=Estados_-_Consumidor."Ler onda - hardware") -> (w423:T5)
        n167 = Enqueue Element(queue=w419, element=w423, error in (no error)=w420) -> (queue out=w418:refnum<queue>, error out=w417:errorcluster)  [unwired: 1 in, 1 out]
      }
    }
    n168 = Or(x=w231, y=w234) -> (x .or. y?=w233:bool)
  }
  n169 = Unregister For Events(event registration refnum=w2) -> ()  [unwired: 1 in, 1 out]
  n170 = Release Queue(queue=w18, error in (no error)=w17) -> (error out=w16:errorcluster)  [unwired: 1 in, 2 out]
  n171 = Merge Errors(w16, w15) -> (w14:errorcluster)
  n172 = call <vilib>:"Simple Error Handler.vi"("error in (no error)"=w14) -> ()  [unwired: 4 in, 5 out]
